vi "CRYCurve Library Interface.vi"(6 "MenuRef":refnum<k9>, 7 "PlatMods":T1, 8 "nButton":u16, 9 "sData":string="XY", 10 "Coords":T2, 11 "sEventName":string="Mouse_Down") -> (3 "bResult":bool)   [LabVIEW 2013]
uses:
  <vilib>/Utility/miscctls.llb/LVPoint32TypeDef.ctl
  CRYWindow/DataView/Control/CRYDrag Graph.ctl
  <vilib>/Utility/miscctls.llb/LVNodeAndColumnTypeDef.ctl
  Global/CRYCurve Library Global.vi
  CRYWindow/DataView/SubVI/CRYData View Global.vi
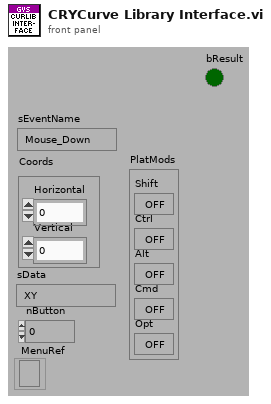
[diagram p1: front panel]
types:
  T1 = cluster{"Shift":bool, "Ctrl":bool, "Alt":bool, "Cmd":bool, "Opt":bool}
  T2 = typedef "LVPoint32TypeDef.ctl" = cluster{"Horizontal":i32, "Vertical":i32}
  T3 = typedef "LVNodeAndColumnTypeDef.ctl" = cluster{"Node":string, "Column":i32}
  T4 = typedef "CRYDrag Graph.ctl" = cluster{"GraphType":string, "GraphData":variant}
  T5 = typedef "CRYCurveLib Info Cluster.ctl" = cluster{"GroupingState":string}
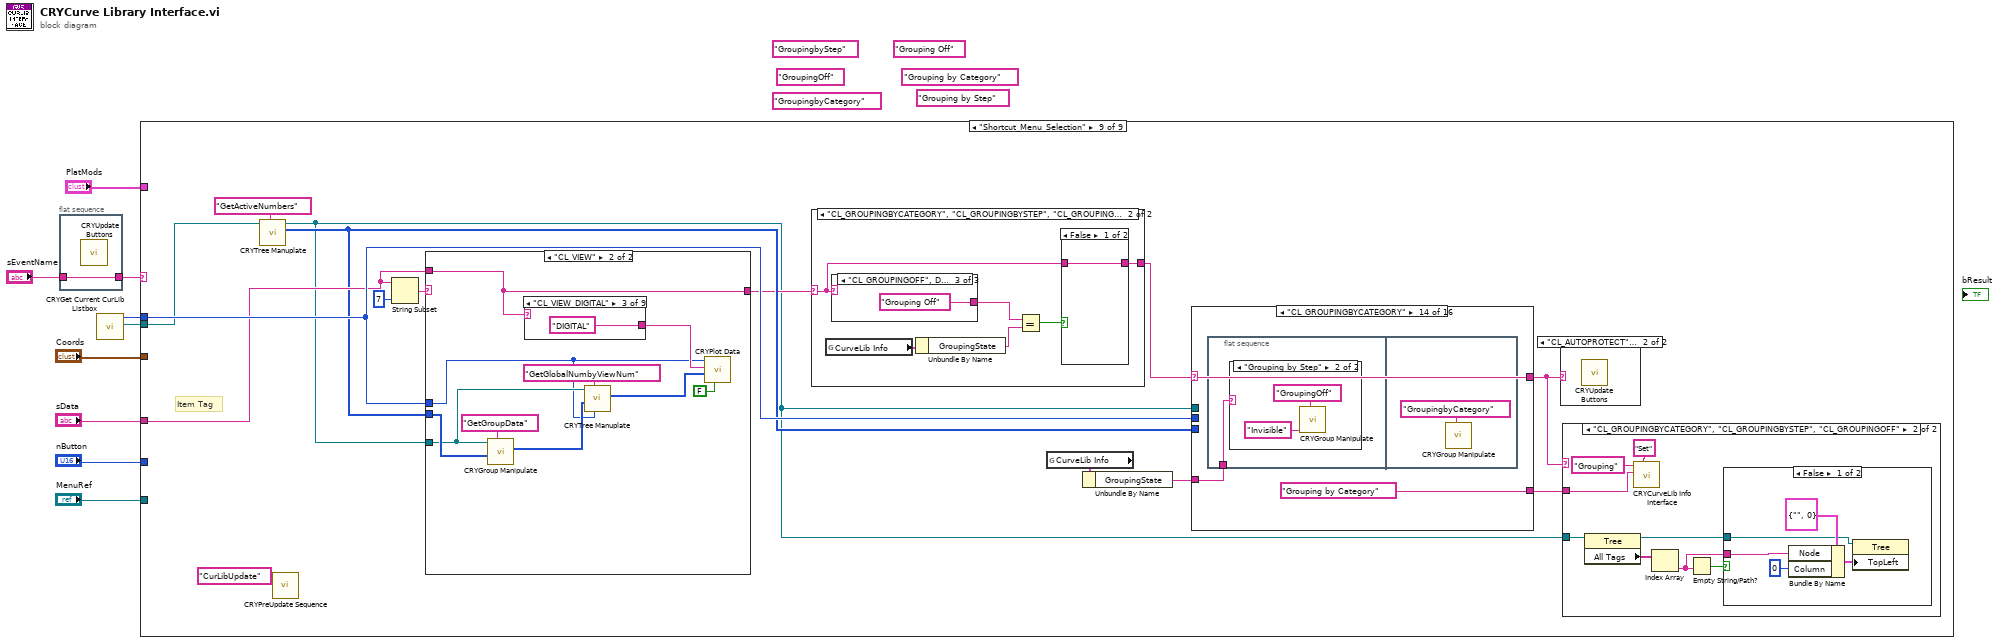
[diagram p0: block diagram]
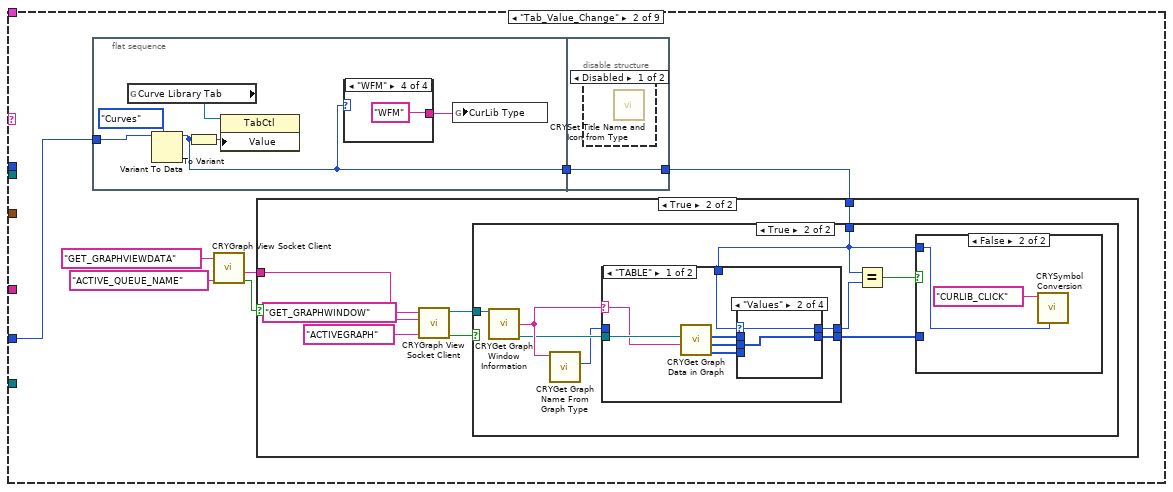
[diagram p3: hidden frame]
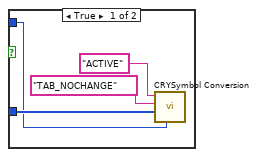
[diagram p6: hidden frame]
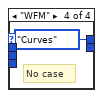
[diagram p9: hidden frame]
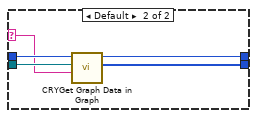
[diagram p10: hidden frame]
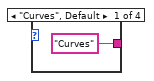
[diagram p11: hidden frame]
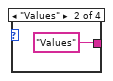
[diagram p12: hidden frame]
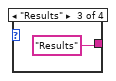
[diagram p13: hidden frame]
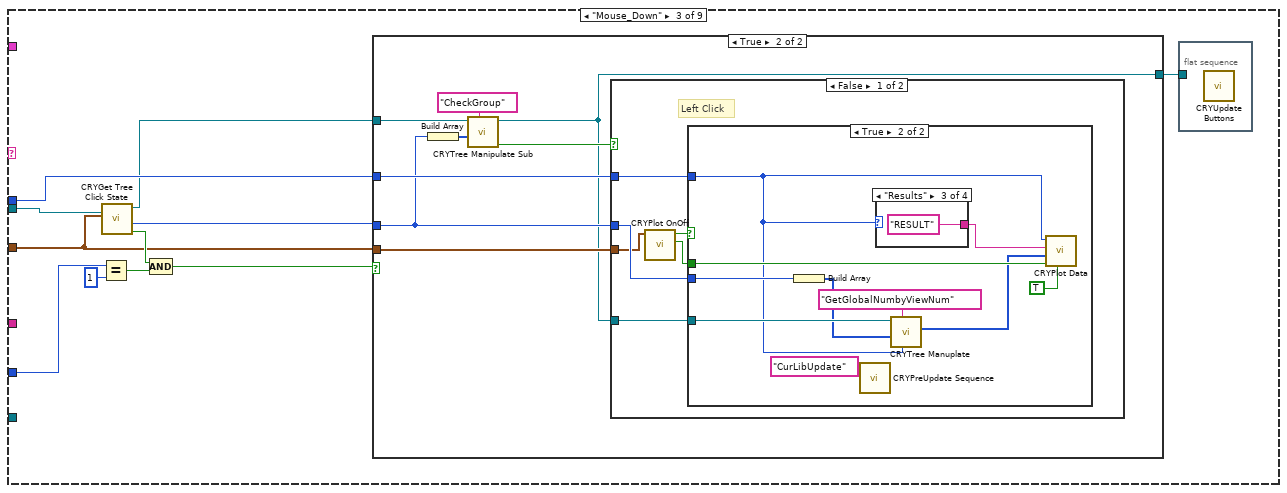
[diagram p15: hidden frame]
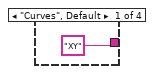
[diagram p18: hidden frame]
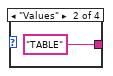
[diagram p19: hidden frame]
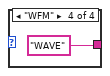
[diagram p20: hidden frame]
diagram:
  (unwired) "Grouping by Step" ("sAction")
  (unwired) "Grouping by Category" ("sAction")
  (unwired) "Grouping Off" ("sAction")
  (unwired) "GroupingbyStep" ("sAction")
  (unwired) "GroupingbyCategory" ("sAction")
  (unwired) "GroupingOff" ("sAction")
  n1 = flat-sequence {
    tunnel: "sEventName" -> [w10]
    tunnel: [w10] -> w2
    frame #0 {
      n2 = call "CRYUpdate Buttons.vi"() -> ()  [unwired: 1 in, 11 out]
    }
  }
  n3 = call "CRYGet Current CurLib Listbox.vi"() -> ("CurLib Tree"=w9:refnum<vi>, "Type"=w8:enum16{"Curves", "Values", "Results", "WFM"})  [unwired: 9 in, 1 out]
  n4 = case shown="\"Shortcut_Menu_Selection\"" w2 {
    tunnel: w9 -> [_ _ w70 w113 w123 w182 w211 w235 w276]
    tunnel: w8 -> [_ _ w77 _ w122 w179 w208 w239 w280]
    tunnel: "nButton" -> [_ w14 w76 w115 w126 _ _ _ _]
    tunnel: "Coords" -> [_ _ w72 w112 _ w180 w212 w237 _]
    tunnel: "sData" -> [_ _ _ _ _ _ w213 _ w279]
    tunnel: "MenuRef" -> [_ _ _ _ _ _ _ w238 _]
    tunnel: "PlatMods" -> [_ _ _ _ w124 _ _ _ _]
    frame Default {
    }
    frame "Tab_Value_Change" {
      n5 = flat-sequence {
        tunnel: w14 -> [w61]
        tunnel: [w58] -> w11
        tunnel: [w68] -> w13
        tunnel: w11 -> [w68]
        frame #0 {
          n6 = global read "CRYCurve Library Global.vi" "Curve Library Tab"() -> (w63:refnum<vi>)
          n7 = Variant To Data(type=enum32{"Curves", "Values", "Results", "WFM"}."Curves" ("Type"), Variant=w61) -> (data=w58:enum32{"Curves", "Values", "Results", "WFM"})  [unwired: 1 in, 1 out]
          n8 = To Variant(anything=w58) -> (Variant=w62:variant)
          n9 = property on="Property Node" class="TabCtl"(reference=w63, "Value"=w62) -> ()  [unwired: 1 in, 2 out]
          n10 = case shown="\"WFM\"" w58 {
            tunnel: ["Curves" "Values" "Results" "WFM"] -> w59
            frame "Curves", Default {
            }
            frame "Values" {
            }
            frame "Results" {
            }
            frame "WFM" {
            }
          }
          n11 = global write "CRYCurve Library Global.vi" "CurLib Type"(w59) -> ()
        }
        frame #1 {
          n12 = disable-structure shown="Disabled" {
            frame Disabled {
              n13 = call "CRYSet Title Name and Icon from Type.vi"() -> ()  [unwired: 12 in]
            }
            frame Enabled {
            }
          }
        }
      }
      n14 = call "CRYGraph View Socket Client.vi"("sOption"="ACTIVE_QUEUE_NAME" ("sAction"), "sAction"="GET_GRAPHVIEWDATA") -> ("bResult Out"=w12:bool, "sData Out"=w15:string)  [unwired: 6 in, 2 out]
      n15 = case shown="True" w12 {
        tunnel: w15 -> [_ w21]
        tunnel: w13 -> [_ w19]
        frame False {
        }
        frame True {
          n16 = call "CRYGraph View Socket Client.vi"("sOption"="ACTIVEGRAPH" ("sAction"), "sData"=w21, "sAction"="GET_GRAPHWINDOW") -> ("bResult Out"=w18:bool, "pVI Out"=w20:refnum<vi>)  [unwired: 5 in, 2 out]
          n17 = case shown="True" w18 {
            tunnel: w20 -> [_ w27]
            tunnel: w19 -> [_ w24]
            frame False {
            }
            frame True {
              n18 = call "CRYGet Graph Window Information.vi"("pGraph VI In"=w27) -> ("Graph Type Out"=w31:string, "Legend Ref Out"=w29:refnum<vi>)  [unwired: 4 in, 9 out]
              n19 = call "CRYGet Graph Name From Graph Type.vi"("Graph Type"=w31) -> ("Type"=w28:enum16{"Curves", "Values", "Results", "WFM"})  [unwired: 9 in, 1 out]
              n20 = case shown="\"TABLE\"" w31 {
                selector: w31 -> [w44 w53]
                tunnel: w28 -> [_ w57]
                tunnel: w29 -> [w45 w56]
                tunnel: [w40 w55] -> w30
                tunnel: [w38 w54] -> w25
                tunnel: w24 -> [w39 _]
                frame "TABLE" {
                  n21 = call "CRYGet Graph Data in Graph.vi"("Graph Type"=w44, "Legend Refnum"=w45) -> ("Result Rows"=w41:i32[], "Value Rows"=w42:i32[], "Rows"=w43:i32[])  [unwired: 2 in, 5 out]
                  n22 = case shown="\"Values\"" w39 {
                    selector: w39 -> [w46 w48 w50 _]
                    tunnel: w43 -> [w47 _ _ _]
                    tunnel: w42 -> [_ w49 _ _]
                    tunnel: w41 -> [_ _ w51 _]
                    tunnel: [w47 w49 w51 _] -> w40
                    tunnel: [w46 w48 w50 enum32{"Curves", "Values", "Results", "WFM"}."Curves" ("Type")] -> w38
                    frame "Curves", Default {
                    }
                    frame "Values" {
                    }
                    frame "Results" {
                    }
                    frame "WFM" {
                      # "No case"
                    }
                  }
                }
                frame Default {
                  n23 = call "CRYGet Graph Data in Graph.vi"("Graph Type"=w53, "Legend Refnum"=w56, "Type In"=w57) -> ("Rows"=w55:i32[], "Type Out"=w54:enum16{"Curves", "Values", "Results", "WFM"})  [unwired: 1 in, 6 out]
                }
              }
              n24 = Equal?(x=w24, y=w25) -> (x = y?=w26:bool)
              n25 = case shown="False" w26 {
                tunnel: w30 -> [w34 _]
                tunnel: w24 -> [w32 w36]
                frame True {
                  n26 = call "CRYSymbol Conversion.vi"("CurLib Tab Type"=w32, "nDatas"=w34, "sData"="TAB_NOCHANGE" ("sActin"), "sActin"="ACTIVE") -> ()  [unwired: 8 in]
                }
                frame False {
                  n27 = call "CRYSymbol Conversion.vi"("CurLib Tab Type"=w36, "sActin"="CURLIB_CLICK") -> ()  [unwired: 10 in]
                }
              }
            }
          }
        }
      }
    }
    frame "Mouse_Down" {
      n28 = Equal?(x=w76, y=u16 1) -> (x = y?=w78:bool)
      n29 = call "CRYGet Tree Click State.vi"("Coords"=w72, "Tree Ref In"=w70) -> ("In Bounds?"=w74:bool, "Row Number"=w73:i32, "Tree Ref Out"=w69:refnum<vi>)  [unwired: 4 in, 3 out]
      n30 = Compound Arithmetic op=AND(w74, w78) -> (w75:bool)
      n31 = case shown="True" w75 {
        tunnel: w72 -> [_ w86]
        tunnel: w73 -> [_ w83]
        tunnel: w77 -> [_ w88]
        tunnel: w69 -> [w80 w84]
        tunnel: [w80 w81] -> w71
        frame False {
        }
        frame True {
          n32 = Build Array(w83) -> (w82:i32[])
          n33 = call "CRYTree Manipulate Sub.vi"("sAction"="CheckGroup", "nData"=w82, "Tree in"=w84) -> ("bData out"=w85:bool, "Tree Out"=w81:refnum<vi>)  [unwired: 4 in, 3 out]
          n34 = case shown="False" w85 {
            tunnel: w83 -> [w92 _]
            tunnel: w88 -> [w91 _]
            tunnel: w86 -> [w90 _]
            tunnel: w81 -> [w89 _]
            frame False {
              # "Left Click"
              n35 = call "CRYPlot OnOff.vi"("Mouse Point"=w90) -> ("Visible?"=w93:bool, "Click State?"=w94:bool)  [unwired: 1 in, 8 out]
              n36 = case shown="True" w94 {
                tunnel: w93 -> [_ w103]
                tunnel: w92 -> [_ w102]
                tunnel: w91 -> [_ w95]
                tunnel: w89 -> [_ w98]
                frame False {
                }
                frame True {
                  n37 = Build Array(w102) -> (w97:i32[])
                  n38 = call "CRYPreUpdate Sequence.vi"("EventName"="CurLibUpdate") -> ()  [unwired: 15 in]
                  n39 = case shown="\"Results\"" w95 {
                    tunnel: ["XY" ("Graph Format") "TABLE" ("Graph Format") "RESULT" ("Graph Format") "WAVE" ("Graph Format")] -> w100
                    frame "Curves", Default {
                    }
                    frame "Values" {
                    }
                    frame "Results" {
                    }
                    frame "WFM" {
                    }
                  }
                  n40 = call "CRYTree Manuplate.vi"("Type"=w95, "sAction"="GetGlobalNumbyViewNum", "nData"=w97, "Tree in"=w98) -> ("nData Out"=w96:i32[])  [unwired: 4 in, 3 out]
                  n41 = call "CRYPlot Data.vi"("Down/Right Click?"=TRUE, "Visible?"=w103, "Rows"=w96, "Graph Type"=w100, "CurLib Tab Type"=w95) -> ()  [unwired: 7 out]
                }
              }
            }
            frame True {
            }
          }
        }
      }
      n42 = flat-sequence {
        tunnel: w71 -> [_]
        frame #0 {
          n43 = call "CRYUpdate Buttons.vi"() -> ()  [unwired: 1 in, 11 out]
        }
      }
    }
    frame "Mouse_Down_Right" {
      n44 = call "CRYGet Tree Click State.vi"("Coords"=w112, "Tree Ref In"=w113) -> ("In Bounds?"=w110:bool, "Row Number"=w109:i32, "Tree Ref Out"=w111:refnum<vi>)  [unwired: 4 in, 3 out]
      n45 = Equal?(x=w115, y=u16 2) -> (x = y?=w117:bool)
      n46 = And(x=w110, y=w117) -> (x .and. y?=w114:bool)
      n47 = case shown="True" w114 {
        tunnel: w109 -> [_ w121]
        tunnel: w111 -> [_ w118]
        frame False {
        }
        frame True {
          # "Right Click"
          n48 = call "CRYGet Selected Rows.vi"("Right Clicked Row"=w121, "Tree Ref In"=w118) -> ("Selected Rows"=w119:i32[])  [unwired: 9 out]
          n49 = call "CRYTree Manuplate.vi"("sAction"="SetActiveNumbers", "nData"=w119, "Tree in"=w118) -> ()  [unwired: 5 in, 4 out]
        }
      }
    }
    frame "Key_Down" {
      n50 = case shown="83" w126 {
        selector: w126 -> [w127 w128 w132 w155 w168 w173]
        tunnel: [w127 w128 w131 w154 w168 w173] -> w125
        tunnel: w124 -> [_ _ _ _ w172 w177]
        tunnel: w123 -> [_ _ w130 w153 _ _]
        tunnel: w122 -> [_ _ w129 _ _ _]
        frame Default {
        }
        frame 72, 80 {
          # "72 up, 80 down"
        }
        frame 83 {
          # "83 - delete"
          n51 = call "CRYUpdate Controls.vi"() -> ("Delete/Rename?"=w133:bool)  [unwired: 1 in, 10 out]
          n52 = case shown="True" w133 {
            tunnel: [u16 0 ("Button") w137] -> w131
            tunnel: w132 -> [_ w137]
            tunnel: w130 -> [_ w136]
            tunnel: w129 -> [_ w135]
            frame False {
            }
            frame True {
              n53 = flat-sequence {
                tunnel: w136 -> [w143]
                tunnel: w135 -> [w140]
                frame #0 {
                  n54 = call "CRYTree Manuplate.vi"("sAction"="GetActiveNumbers", "Tree in"=w143) -> ("nData Out"=w146:i32[], "Tree Out"=w145:refnum<vi>)  [unwired: 6 in, 2 out]
                  n55 = call "CRYTree Manipulate Sub.vi"("sAction"="CheckGroup", "nData"=w146, "Tree in"=w145) -> ("bOnlyGroup"=w139:bool, "Tree Out"=w142:refnum<vi>, "bCategory"=w138:bool)  [unwired: 4 in, 2 out]
                  n56 = case shown="False" w138 {
                    tunnel: w142 -> [w149 _]
                    tunnel: w140 -> [w148 _]
                    tunnel: w139 -> [w147 _]
                    frame False {
                      n57 = case shown="True" w147 {
                        tunnel: w149 -> [_ w151]
                        tunnel: w148 -> [_ w150]
                        frame False {
                          n58 = call "CRYDelete All.vi"() -> ()  [unwired: 3 in, 9 out]
                        }
                        frame True {
                          n59 = call "CRYGroup Manipulate.vi"("sAction"="DeleteGroupData", "Type"=w150, "Tree in"=w151) -> ()  [unwired: 5 in, 4 out]
                        }
                      }
                    }
                    frame True {
                    }
                  }
                }
                frame #1 {
                  n60 = call "CRYUpdate Steps Input Control.vi"() -> ()  [unwired: 12 in]
                }
              }
            }
          }
        }
        frame 60 {
          # "60 - rename"
          n61 = call "CRYUpdate Controls.vi"() -> ("Save/Export?"=w156:bool)  [unwired: 1 in, 10 out]
          n62 = case shown="True" w156 {
            tunnel: [u16 0 ("Button") w165] -> w154
            tunnel: w155 -> [_ w165]
            tunnel: w153 -> [_ w158]
            frame False {
            }
            frame True {
              n63 = call "CRYTree Manuplate.vi"("sAction"="GetActiveNumbers", "Tree in"=w158) -> ("nData Out"=w159:i32[], "Tree Out"=w160:refnum<vi>)  [unwired: 6 in, 2 out]
              n64 = call "CRYTree Manipulate Sub.vi"("sAction"="CheckGroup", "nData"=w159, "Tree in"=w160) -> ("bData out"=w162:bool, "Tree Out"=w163:refnum<vi>)  [unwired: 4 in, 3 out]
              n65 = case shown="False" w162 {
                tunnel: w163 -> [_ w166]
                frame False {
                  n66 = call "CRYRename All.vi"() -> ()  [unwired: 1 in, 11 out]
                }
                frame True {
                  n67 = call "CRYGroup Manipulate.vi"("sAction"="Rename", "Tree in"=w166) -> ()  [unwired: 6 in, 4 out]
                }
              }
            }
          }
        }
        frame 88 {
          # "Ctrl+F12-> Complete Delete by Index"
          n68 = Unbundle By Name(w172) -> ("Opt"=w170:bool, "Ctrl"=w171:bool)
          n69 = And(x=w170, y=w171) -> (x .and. y?=w169:bool)
          n70 = case shown="True" w169 {
            frame False {
            }
            frame True {
              n71 = flat-sequence {
                frame #0 {
                  n72 = call "CRYDelete All Complete.vi"() -> ()  [unwired: 10 in, 2 out]
                }
                frame #1 {
                  n73 = call "CRYUpdate Steps Input Control.vi"() -> ()  [unwired: 12 in]
                }
              }
            }
          }
        }
        frame 87 {
          # "Ctrl+F11-> Complete Delete All"
          n74 = Unbundle By Name(w177) -> ("Opt"=w175:bool, "Ctrl"=w176:bool)
          n75 = And(x=w175, y=w176) -> (x .and. y?=w174:bool)
          n76 = case shown="True" w174 {
            frame False {
            }
            frame True {
              n77 = flat-sequence {
                frame #0 {
                  n78 = call "CRYDelete All Complete.vi"("sAction"="All") -> ()  [unwired: 9 in, 2 out]
                }
                frame #1 {
                  n79 = call "CRYUpdate Steps Input Control.vi"() -> ()  [unwired: 12 in]
                }
              }
            }
          }
        }
      }
      n80 = case shown="60, 83" w125 {
        frame Default {
        }
        frame 60, 83 {
          n81 = call "CRYUpdate Buttons.vi"() -> ()  [unwired: 1 in, 11 out]
        }
      }
    }
    frame "Double_Click" {
      # "Click Name Only ?"
      n82 = call "CRYGet Tree Click State.vi"("Coords"=w180, "Tree Ref In"=w182) -> ("In Bounds?"=w184:bool, "Row Number"=w185:i32, "Tree Ref Out"=w181:refnum<vi>, "In Symbol?"=w183:bool)  [unwired: 4 in, 2 out]
      n83 = case shown="\"Curves\", Default" w179 {
        tunnel: ["Probe Curve" ("WindowType") "Probe Value" ("WindowType") "Probe Result" ("WindowType") "Probe Waveform" ("WindowType")] -> w187
        frame "Curves", Default {
        }
        frame "Values" {
        }
        frame "Results" {
        }
        frame "WFM" {
        }
      }
      n84 = Compound Arithmetic op=AND(w184, invert w183) -> (w186:bool)
      n85 = case shown="True" w186 {
        tunnel: w185 -> [_ w195]
        tunnel: w187 -> [_ w199]
        tunnel: w181 -> [_ w196]
        tunnel: w179 -> [_ w192]
        frame False {
        }
        frame True {
          n86 = Build Array(w195) -> (w194:i32[])
          n87 = call "CRYTree Manipulate Sub.vi"("sAction"="CheckGroup", "nData"=w194, "Tree in"=w196) -> ("bData out"=w197:bool, "Tree Out"=w193:refnum<vi>)  [unwired: 4 in, 3 out]
          n88 = case shown="False" w197 {
            tunnel: w195 -> [w203 _]
            tunnel: w199 -> [w207 _]
            tunnel: w193 -> [w201 _]
            tunnel: w192 -> [w200 _]
            frame False {
              n89 = Build Array(w203) -> (w205:i32[])
              n90 = call "CRYTree Manuplate.vi"("Type"=w200, "sAction"="GetGlobalNumbyViewNum", "nData"=w205, "Tree in"=w201) -> ("nData Out"=w204:i32[])  [unwired: 4 in, 3 out]
              n91 = Index Array(array=w204) -> (element=w202:i32)  [unwired: 1 in]
              n92 = call "CRYProbe Window Display.vi"("Row"=w202, "Probe Type"=w207) -> ()  [unwired: 10 out]
            }
            frame True {
            }
          }
        }
      }
    }
    frame "Drag_Starting" {
      # "GraphType"
      n93 = call "CRYGet Tree Click State.vi"("Coords"=w212, "Tree Ref In"=w211) -> ("In Bounds?"=w209:bool, "Tree Ref Out"=w210:refnum<vi>)  [unwired: 4 in, 4 out]
      n94 = case shown="True" w209 {
        tunnel: w210 -> [_ w222]
        tunnel: w213 -> [_ w230]
        tunnel: w208 -> [_ w220]
        frame False {
        }
        frame True {
          w231 = T4 {"GraphType"="", "GraphData"=variant}  # Drag Graph Cluster
          n95 = property class="Tree"(reference=w222) -> ("Value"=w225:variant)  [unwired: 1 in, 2 out]
          n96 = call "CRYTree Manuplate.vi"("sAction"="GetActiveNumbers", "Tree in"=w222) -> ("nData Out"=w215:i32[], "Tree Out"=w217:refnum<vi>)  [unwired: 6 in, 2 out]
          n97 = Bundle By Name(cluster=cluster{"DataName":string, "DragData":variant} {"DataName"="", "DragData"=variant} ("Drag into CurLib"), "DataName"="CRY_CURLIB_DATA" ("data name"), "DragData"=w225) -> (w226:cluster{"DataName":string, "DragData":variant})
          n98 = call "CRYGroup Manipulate.vi"("sAction"="GetDragData", "nData"=w215, "Tree in"=w217) -> ("nData Out"=w214:i32[], "Tree Out"=w216:refnum<vi>)  [unwired: 5 in, 2 out]
          n99 = global write "CRYCurve Library Global.vi" "Drag into CurLib"(w226) -> ()
          n100 = Sort 1D Array(array=w214) -> (sorted array=w219:i32[])
          n101 = call "CRYTree Manuplate.vi"("Type"=w220, "sAction"="GetGlobalNumbyViewNum", "nData"=w219, "Tree in"=w216) -> ("nData Out"=w221:i32[])  [unwired: 4 in, 3 out]
          n102 = Bundle By Name(cluster=w231, "GraphType"=w230, "GraphData"=w221) -> (w228:T4)
          n103 = global write "CRYData View Global.vi" "Drag into Graph"(w228) -> ()
        }
      }
    }
    frame "Shortcut_Menu_Activation" {
      n104 = call "CRYGet Tree Click State.vi"("Coords"=w237, "Tree Ref In"=w235) -> ("In Bounds?"=w234:bool, "Row Number"=w232:i32, "Tree Ref Out"=w233:refnum<vi>)  [unwired: 4 in, 3 out]
      n105 = case shown="True" w234 {
        selector: w234 -> [w240 _]
        tunnel: w239 -> [_ w252]
        tunnel: w238 -> [w241 w251]
        tunnel: [w240 w249] -> w236
        tunnel: w233 -> [_ w243]
        tunnel: w232 -> [_ _]
        frame False {
          n106 = Delete Menu Items(9:w241) -> ()  [unwired: 2 in, 3 out]
        }
        frame True {
          n107 = call "CRYTree Manuplate.vi"("sAction"="GetActiveNumbers", "Tree in"=w243) -> ("nData Out"=w245:i32[], "Tree Out"=w246:refnum<vi>)  [unwired: 6 in, 2 out]
          n108 = call "CRYTree Manuplate.vi"("sAction"="GetActiveTags", "Tree in"=w243) -> ("sData Out"=w242:string[])  [unwired: 6 in, 3 out]
          n109 = call "CRYTree Manipulate Sub.vi"("sAction"="CheckCombineGroupandData", "nData"=w245, "Tree in"=w246) -> ("bData out"=w249:bool, "Tree Out"=w248:refnum<vi>)  [unwired: 4 in, 3 out]
          n110 = case shown="False" w249 {
            tunnel: w252 -> [w268 _]
            tunnel: w251 -> [w267 _]
            tunnel: w245 -> [w263 _]
            tunnel: w248 -> [w262 _]
            tunnel: w242 -> [w261 _]
            frame False {
              n111 = Index Array(array=w261) -> (element=w260:string)  [unwired: 1 in]
              n112 = invoke class="Tree" method="Navigate Tree.Get Parent"(reference=w262, "tag"=w260) -> (reference out=w256:refnum<vi>, "Navigate Tree:Get Parent"=w258:string)  [unwired: 2 in, 2 out]
              n113 = Build Array(w258) -> (w257:string[])
              n114 = call "CRYTree Manipulate Sub.vi"("sAction"="CheckGroup", "sData"=w257, "sOption"="byTag", "Tree in"=w256) -> ("bCategory"=w254:bool)  [unwired: 3 in, 4 out]
              n115 = call "CRYTree Manipulate Sub.vi"("sAction"="CheckGroup", "nData"=w263, "Tree in"=w256) -> ("bData out"=w265:bool, "bCategory"=w255:bool)  [unwired: 4 in, 3 out]
              n116 = Or(x=w255, y=w254) -> (x .or. y?=w253:bool)
              n117 = call "CRYCurve Library Popup Menu.vi"("Category?"=w253, "Group?"=w265, "Type"=w268, "Menu Ref In"=w267) -> ()  [unwired: 8 out]
            }
            frame True {
            }
          }
        }
      }
      n118 = local write "bResult"(w236) -> ()
    }
    frame "Shortcut_Menu_Selection" {
      # "Item Tag"
      n119 = call "CRYTree Manuplate.vi"("sAction"="GetActiveNumbers", "Tree in"=w276) -> ("nData Out"=w277:i32[], "Tree Out"=w269:refnum<vi>)  [unwired: 6 in, 2 out]
      n120 = call "CRYPreUpdate Sequence.vi"("EventName"="CurLibUpdate") -> ()  [unwired: 15 in]
      n121 = String Subset(string=w279, length (rest)=7 ("length (rest)")) -> (substring=w281:string)  [unwired: 1 out]
      n122 = case shown="\"CL_VIEW\"" w281 {
        tunnel: [w309 w319] -> w273
        tunnel: w280 -> [_ w310]
        tunnel: w277 -> [_ w312]
        tunnel: w279 -> [w309 w319]
        tunnel: w269 -> [_ w311]
        frame Default {
        }
        frame "CL_VIEW" {
          n123 = call "CRYGroup Manipulate.vi"("sAction"="GetGroupData", "nData"=w312, "Tree in"=w311) -> ("nData Out"=w313:i32[])  [unwired: 5 in, 3 out]
          n124 = case shown="\"CL_VIEW_DIGITAL\"" w319 {
            selector: w319 -> [_ _ _ _ _ _ _ _ w328]
            tunnel: ["XY" ("Graph Format") "OCTAVE" ("Graph Format") "DIGITAL" ("Graph Format") "POLAR" ("Graph Format") "WAVE" ("Graph Format") "INTENSITY" ("Graph Format") "TABLE" ("Graph Format") "RESULT" ("Graph Format") w328] -> w317
            frame "CL_VIEW_XY" {
            }
            frame "CL_VIEW_OCTAVE" {
            }
            frame "CL_VIEW_DIGITAL" {
            }
            frame "CL_VIEW_POLAR" {
            }
            frame "CL_VIEW_WAVE" {
            }
            frame "CL_VIEW_INTENSITY" {
            }
            frame "CL_VIEW_TABLE" {
            }
            frame "CL_VIEW_RESULT" {
            }
            frame "CL_VIEW_TEXT", Default {
            }
          }
          n125 = call "CRYTree Manuplate.vi"("Type"=w310, "sAction"="GetGlobalNumbyViewNum", "nData"=w313, "Tree in"=w311) -> ("nData Out"=w315:i32[])  [unwired: 4 in, 3 out]
          n126 = call "CRYPlot Data.vi"("Down/Right Click?"=FALSE, "Rows"=w315, "Graph Type"=w317, "CurLib Tab Type"=w310) -> ()  [unwired: 1 in, 7 out]
        }
      }
      n127 = case shown="\"CL_GROUPINGBYCATEGORY\", \"CL_GROUPINGBYSTEP\", \"CL_GROUPINGOFF\"" w273 {
        selector: w273 -> [w284 w286]
        tunnel: [w284 w285] -> w272
        frame Default {
        }
        frame "CL_GROUPINGBYCATEGORY", "CL_GROUPINGBYSTEP", "CL_GROUPINGOFF" {
          n128 = global read "CRYCurve Library Global.vi" "CurveLib Info"() -> (w290:T5)
          n129 = case shown="\"CL_GROUPINGOFF\", Default" w286 {
            tunnel: ["Grouping by Category" ("sAction") "Grouping by Step" ("sAction") "Grouping Off" ("sAction")] -> w289
            frame "CL_GROUPINGBYCATEGORY" {
            }
            frame "CL_GROUPINGBYSTEP" {
            }
            frame "CL_GROUPINGOFF", Default {
            }
          }
          n130 = Unbundle By Name(w290) -> ("GroupingState"=w288:string)
          n131 = Equal?(x=w289, y=w288) -> (x = y?=w287:bool)
          n132 = case shown="False" w287 {
            tunnel: w286 -> [w291 _]
            tunnel: [w291 "None"] -> w285
            frame False {
            }
            frame True {
            }
          }
        }
      }
      n133 = global read "CRYCurve Library Global.vi" "CurveLib Info"() -> (w271:T5)
      n134 = Unbundle By Name(w271) -> ("GroupingState"=w270:string)
      n135 = case shown="\"CL_GROUPINGBYCATEGORY\"" w272 {
        selector: w272 -> [w329 w330 w331 w332 w333 w342 w343 w351 w359 w362 w365 w372 w375 w378 w385 w390]
        tunnel: w277 -> [_ _ _ _ _ w337 _ w346 _ _ _ _ _ _ _ _]
        tunnel: [w329 w330 w331 w332 w333 w342 w343 w351 w359 w362 w365 w372 w375 w378 w385 w390] -> w275
        tunnel: w280 -> [_ _ _ _ _ w339 _ w344 w356 _ w363 w369 _ _ _ _]
        tunnel: w269 -> [_ _ _ _ _ w335 _ w347 w357 w360 w364 w370 _ _ _ _]
        tunnel: [_ _ _ _ _ _ _ _ _ _ _ _ "Grouping Off" ("sAction") "Grouping by Category" ("sAction") "Grouping by Step" ("sAction") _] -> w274
        tunnel: w270 -> [_ _ _ _ _ _ _ _ _ _ _ _ _ w376 w383 _]
        frame "CL_PROTECT" {
          n136 = call "CRYProtect All.vi"() -> ()  [unwired: 4 in, 8 out]
        }
        frame "CL_AUTOPROTECT" {
          n137 = call "CRYAutoProtect All.vi"() -> ()  [unwired: 10 in, 2 out]
        }
        frame "CL_AUTOUNPROTECT" {
          n138 = call "CRYUndo AutoProtect.vi"() -> ()  [unwired: 12 out]
        }
        frame "CL_DELETE" {
          n139 = flat-sequence {
            frame #0 {
              n140 = call "CRYDelete All.vi"() -> ()  [unwired: 3 in, 9 out]
            }
            frame #1 {
              n141 = call "CRYUpdate Steps Input Control.vi"() -> ()  [unwired: 12 in]
            }
          }
        }
        frame "CL_RENAME" {
          n142 = call "CRYRename All.vi"() -> ()  [unwired: 1 in, 11 out]
        }
        frame "CL_EXPORT_EXCEL" {
          n143 = call "CRYGroup Manipulate.vi"("sAction"="GetGroupData", "nData"=w337, "Tree in"=w335) -> ("nData Out"=w336:i32[], "Tree Out"=w334:refnum<vi>)  [unwired: 5 in, 2 out]
          n144 = call "CRYTree Manuplate.vi"("Type"=w339, "sAction"="GetGlobalNumbyViewNum", "nData"=w336, "Tree in"=w334) -> ("nData Out"=w340:i32[])  [unwired: 4 in, 3 out]
          n145 = call "CRYExport to Excel.vi"("Rows"=w340, "Type"=w339) -> ()  [unwired: 2 in, 8 out]
        }
        frame "CL_IMPORT_TEXT" {
          n146 = call "CRYImport From File.vi"() -> ()  [unwired: 12 in]
        }
        frame "CL_PROBE" {
          n147 = case shown="\"Curves\", Default" w344 {
            tunnel: ["Probe Curve" ("WindowType") "Probe Value" ("WindowType") "Probe Result" ("WindowType") "Probe Waveform" ("WindowType")] -> w350
            frame "Curves", Default {
            }
            frame "Values" {
            }
            frame "Results" {
            }
            frame "WFM" {
            }
          }
          n148 = call "CRYTree Manuplate.vi"("Type"=w344, "sAction"="GetGlobalNumbyViewNum", "nData"=w346, "Tree in"=w347) -> ("nData Out"=w345:i32[])  [unwired: 4 in, 3 out]
          n149 = Index Array(array=w345) -> (element=w349:i32)  [unwired: 1 in]
          n150 = call "CRYProbe Window Display.vi"("Row"=w349, "Probe Type"=w350) -> ()  [unwired: 10 out]
        }
        frame "CL_NEWGROUP" {
          n151 = call "CRYGroup Manipulate.vi"("sAction"="NewGroup", "Type"=w356, "Tree in"=w357) -> ()  [unwired: 5 in, 4 out]
        }
        frame "CL_UNGROUP" {
          n152 = call "CRYGroup Manipulate.vi"("sAction"="UnGroup", "Tree in"=w360) -> ()  [unwired: 6 in, 4 out]
        }
        frame "CL_DELETEGROUPDATA" {
          n153 = flat-sequence {
            tunnel: w364 -> [w367]
            tunnel: w363 -> [w366]
            frame #0 {
              n154 = call "CRYGroup Manipulate.vi"("sAction"="DeleteGroupData", "Type"=w366, "Tree in"=w367) -> ()  [unwired: 5 in, 4 out]
            }
            frame #1 {
              n155 = call "CRYUpdate Steps Input Control.vi"() -> ()  [unwired: 12 in]
            }
          }
        }
        frame "CL_RENAMEGROUP" {
          n156 = call "CRYGroup Manipulate.vi"("sAction"="Rename", "Type"=w369, "Tree in"=w370) -> ()  [unwired: 5 in, 4 out]
        }
        frame "CL_GROUPINGOFF" {
          n157 = call "CRYGroup Manipulate.vi"("sAction"="GroupingOff") -> ()  [unwired: 7 in, 4 out]
        }
        frame "CL_GROUPINGBYCATEGORY" {
          n158 = flat-sequence {
            tunnel: w376 -> [w379]
            frame #0 {
              n159 = case shown="\"Grouping by Step\"" w379 {
                frame "GroupingOff", Default {
                }
                frame "Grouping by Step" {
                  n160 = call "CRYGroup Manipulate.vi"("sAction"="GroupingOff", "sOption"="Invisible") -> ()  [unwired: 6 in, 4 out]
                }
              }
            }
            frame #1 {
              n161 = call "CRYGroup Manipulate.vi"("sAction"="GroupingbyCategory") -> ()  [unwired: 7 in, 4 out]
            }
          }
        }
        frame "CL_GROUPINGBYSTEP" {
          n162 = flat-sequence {
            tunnel: w383 -> [w386]
            frame #0 {
              n163 = case shown="\"Grouping by Category\"" w386 {
                frame "GroupingOff", Default {
                }
                frame "Grouping by Category" {
                  n164 = call "CRYGroup Manipulate.vi"("sAction"="GroupingOff", "sOption"="Invisible") -> ()  [unwired: 6 in, 4 out]
                }
              }
            }
            frame #1 {
              n165 = call "CRYGroup Manipulate.vi"("sAction"="GroupingbyStep") -> ()  [unwired: 7 in, 4 out]
            }
          }
        }
        frame "None", Default {
        }
      }
      n166 = case shown="\"CL_AUTOPROTECT\", \"CL_AUTOUNPROTECT\", \"CL_DELETE\", \"CL_PROTECT\"" w275 {
        frame Default {
        }
        frame "CL_AUTOPROTECT", "CL_AUTOUNPROTECT", "CL_DELETE", "CL_PROTECT" {
          n167 = call "CRYUpdate Buttons.vi"() -> ()  [unwired: 1 in, 11 out]
        }
      }
      n168 = case shown="\"CL_GROUPINGBYCATEGORY\", \"CL_GROUPINGBYSTEP\", \"CL_GROUPINGOFF\"" w275 {
        tunnel: w274 -> [_ w301]
        tunnel: w269 -> [_ w300]
        frame Default {
        }
        frame "CL_GROUPINGBYCATEGORY", "CL_GROUPINGBYSTEP", "CL_GROUPINGOFF" {
          n169 = property class="Tree"(reference=w300) -> (reference out=w296:refnum<vi>, "All Tags"=w299:string[])  [unwired: 1 in, 1 out]
          n170 = call "CRYCurveLib Info Interface.vi"("sAction"="Set", "sData"=w301, "sOption"="Grouping" ("Key")) -> ()  [unwired: 9 in]
          n171 = Index Array(array=w299) -> (element=w297:string)  [unwired: 1 in]
          n172 = Empty String/Path?(string/path=w297) -> (empty?=w298:bool)
          n173 = case shown="False" w298 {
            tunnel: w297 -> [w305 _]
            tunnel: w296 -> [w304 _]
            frame False {
              n174 = Bundle By Name(cluster=T3 {"Node"="", "Column"=0} ("Top Left Visible Cell"), "Node"=w305, "Column"=0) -> (w307:T3)
              n175 = property class="Tree"(reference=w304, "TopLeft"=w307) -> ()  [unwired: 1 in, 2 out]
            }
            frame True {
            }
          }
        }
      }
    }
  }
